vi "_087.vi"() -> ()   [LabVIEW 2024]
panel:
  out "Array 3":i32[](array[numeric])
  out "appended array":i32[](array[numeric])
  out "element":i32
  out "Array 2":i32[](array[numeric])
  out "Array":i32[](array[numeric])
  # "Fundamentals :"
  # "16~>After running this VI,what is the value displayed in the o/p & iteration count?"
  # "Nrml Approach :"
  # "Dfrnt Approach :"
  # "( Work flow )"
  # "The loop will run based on the array size. The Array Size is 3 the loop will be run 3times. The WorkFlow of the loop is the sum (element values) of build array + each element of the array."
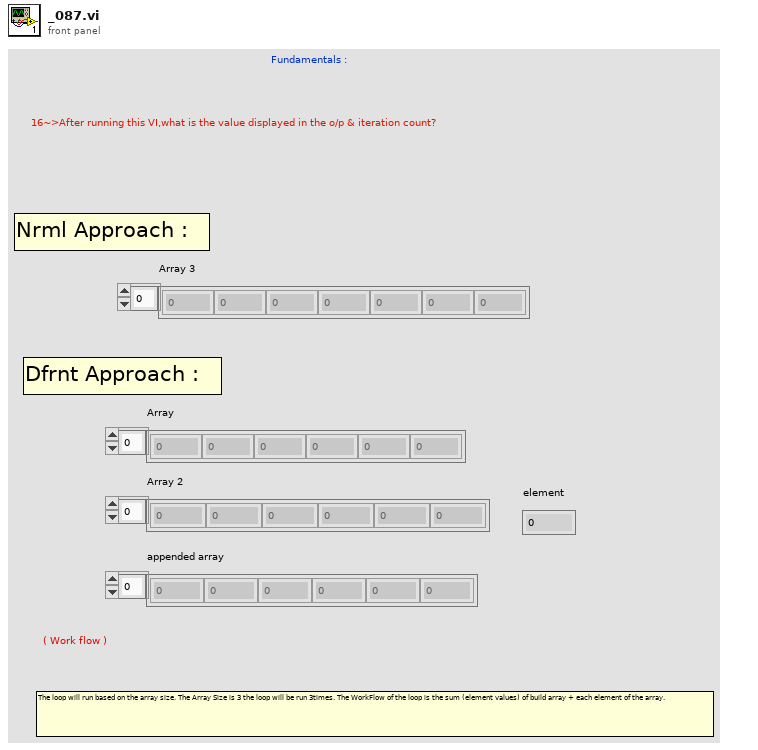
[diagram p1: front panel]
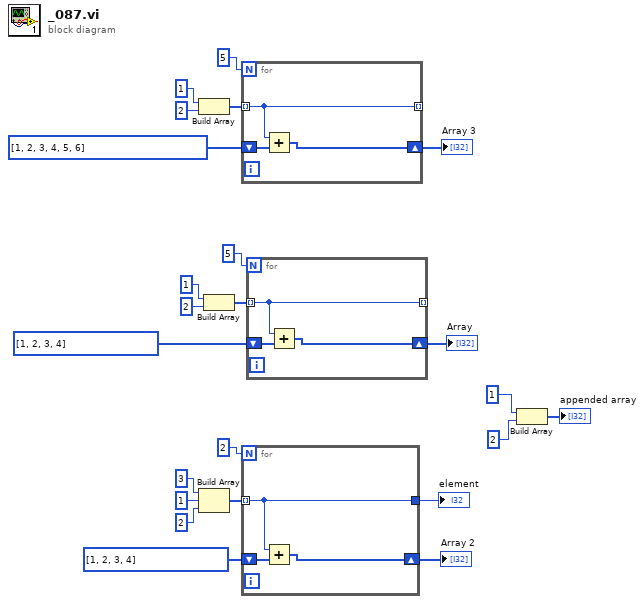
[diagram p0: block diagram]
diagram:
  n1 = Build Array(1, 2) -> (w3:i32[])
  n2 = Build Array "Build Array"(3 ("element"), 1, 2) -> (w14:i32[])
  n3 = Build Array(1, 2) -> (w21:i32[])
  n4 = for {
    N: 5 -> [_]
    tunnel: [w26] -> _ mode=indexing
    tunnel: w3 -> [w26] mode=indexing
    shift-right: [w24] -> w6
    shift-left: i32[] [1, 2, 3, 4, 5, 6] -> [w25]
    n5 = Add(x=w26, y=w25) -> (x+y=w24:i32[])
  }
  "Array 3" <- w6
  n6 = for {
    N: 2 -> [_]
    tunnel: [w29] -> w10
    tunnel: w14 -> [w29] mode=indexing
    shift-right: [w28] -> w17
    shift-left: i32[] [1, 2, 3, 4] -> [w27]
    n7 = Add(x=w29, y=w27) -> (x+y=w28:i32[])
  }
  "Array 2" <- w17
  "element" <- w10
  n8 = for {
    N: 5 -> [_]
    tunnel: [w32] -> _ mode=indexing
    tunnel: w21 -> [w32] mode=indexing
    shift-right: [w30] -> w18
    shift-left: i32[] [1, 2, 3, 4] -> [w31]
    n9 = Add(x=w32, y=w31) -> (x+y=w30:i32[])
  }
  "Array" <- w18
  n10 = Build Array(1, 2) -> (→"appended array":i32[])
